vi "Layout FGV.vi"(7 "String":string, 8 "error in (no error)":errorcluster, 11 "InitRef":T5) -> (0 "error out":errorcluster)   [LabVIEW 2020, in "MDI ViewManager.lvlib"]
uses:
  MDI ViewManager.lvlib
  <vilib>/Utility/miscctls.llb/LVPositionTypeDef.ctl
  <vilib>/Utility/miscctls.llb/LVBoundsTypeDef.ctl
  <vilib>/Utility/miscctls.llb/LVPointTypeDef.ctl
  Typedef/Update ViewList.ctl
  Typedef/LayoutMap.ctl
panel:
  in  "map in":map{string, T1}(c390)
  in  "Variant":variant
  in  "name":string
  in  "file (use dialog)":path
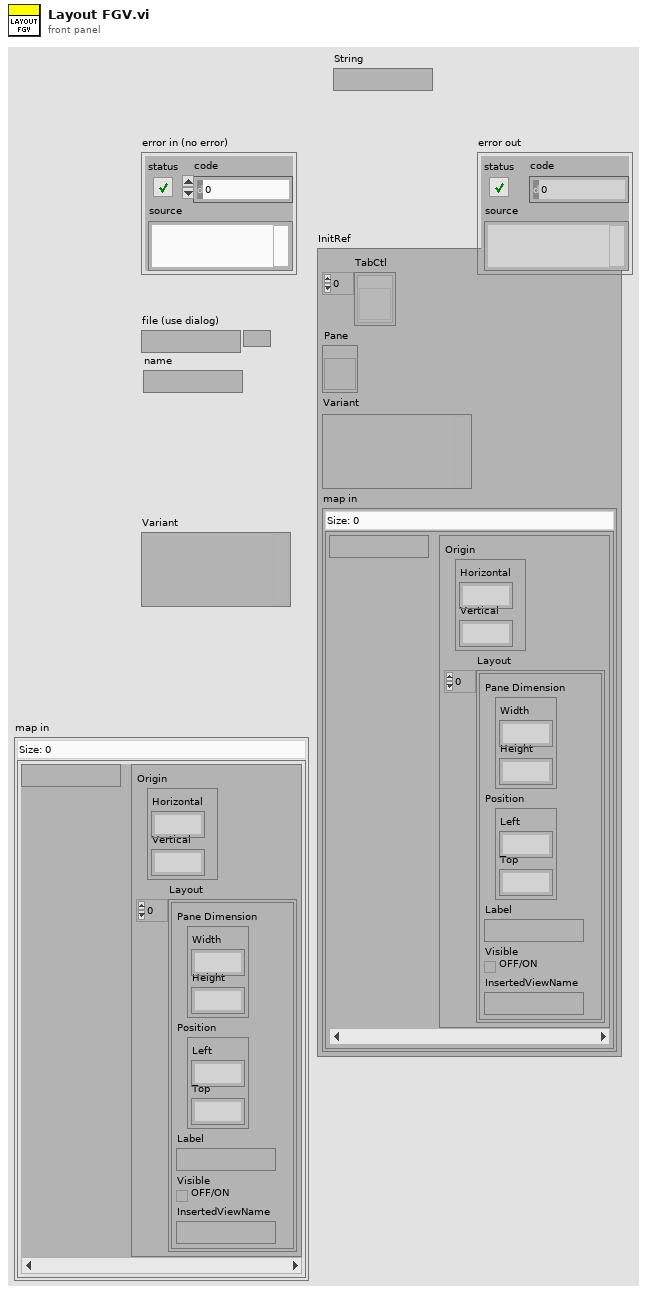
[diagram p1: front panel]
types:
  T1 = typedef "MDI ViewManager.lvlib/LayoutMap.ctl" = cluster{"Origin":T2, "Layout":cluster{"Pane Dimension":T3, "Position":T4, "Label":string, "Visible":bool, "InsertedViewName":string}[]}
  T2 = typedef "LVPointTypeDef.ctl" = cluster{"Horizontal":i16, "Vertical":i16}
  T3 = typedef "LVBoundsTypeDef.ctl" = cluster{"Width":u32, "Height":u32}
  T4 = typedef "LVPositionTypeDef.ctl" = cluster{"Left":i32, "Top":i32}
  T5 = cluster{"TabCtl":refnum<vi>[], "Pane":refnum<vi>, "Variant":variant, "map in":map{string, T1}}
  T6 = cluster{"Origin":T2, "Layout":cluster{"Pane Dimension":T3, "Position":T4, "Label":string, "Visible":bool, "InsertedViewName":string}[]}
  T7 = typedef "MDI ViewManager.lvlib/Update ViewList.ctl" = cluster{"Name":string, "VIPath":path, "Height(Default)":u32, "Widht(Default)":u32, "VIRef":refnum<vi>}
  T8 = cluster{"Pane Dimension":T3, "Position":T4, "Label":string, "Visible":bool, "InsertedViewName":string}
  T9 = cluster{"Pane Dimension":T3, "Position":T4, "Label":string, "Visible":bool, "InsertedViewName":string}[]
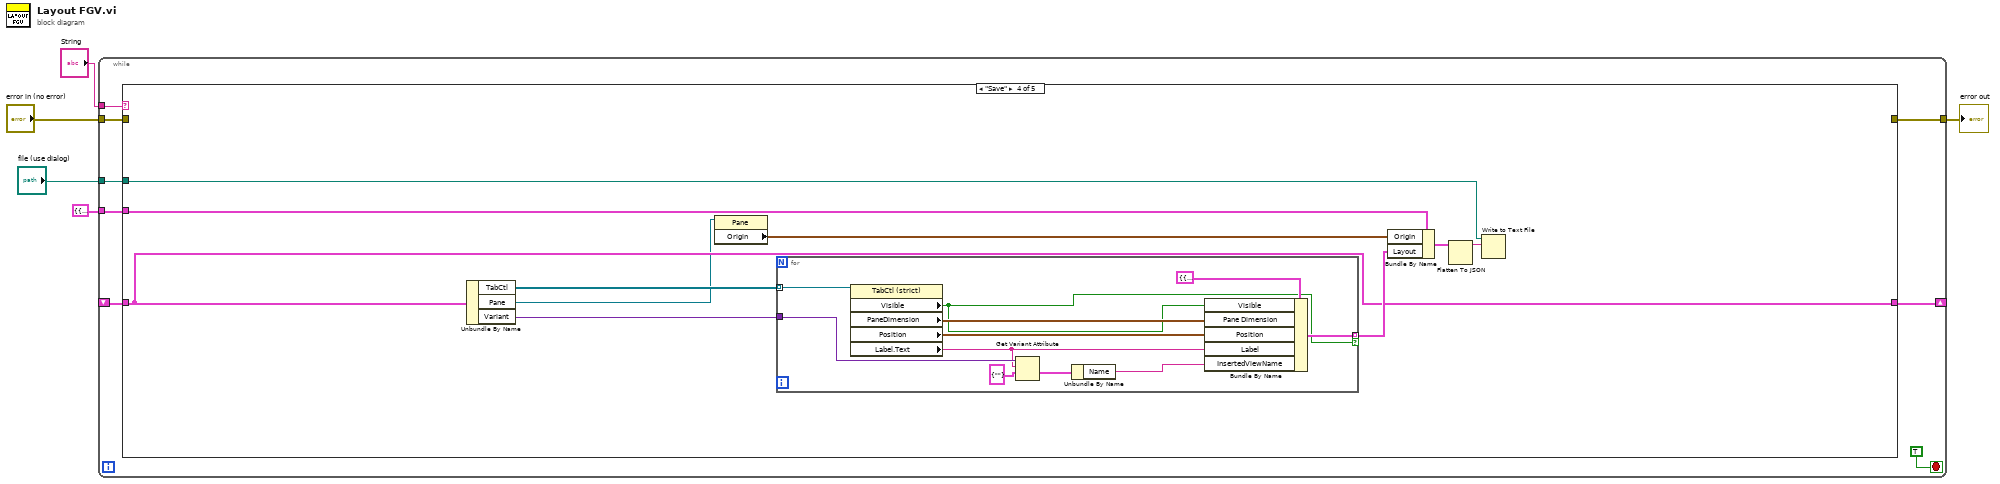
[diagram p0: block diagram]
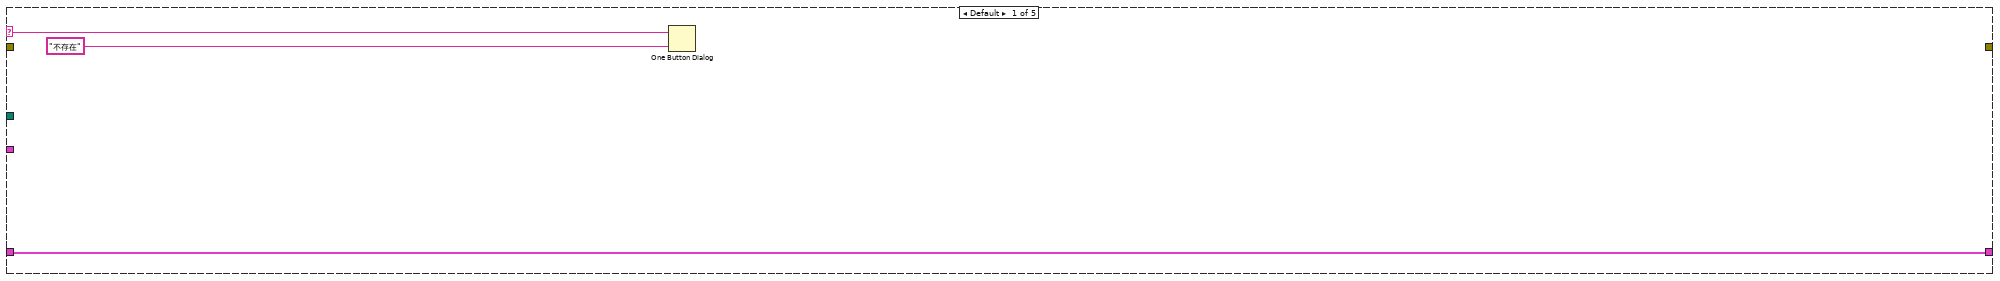
[diagram p2: hidden frame]
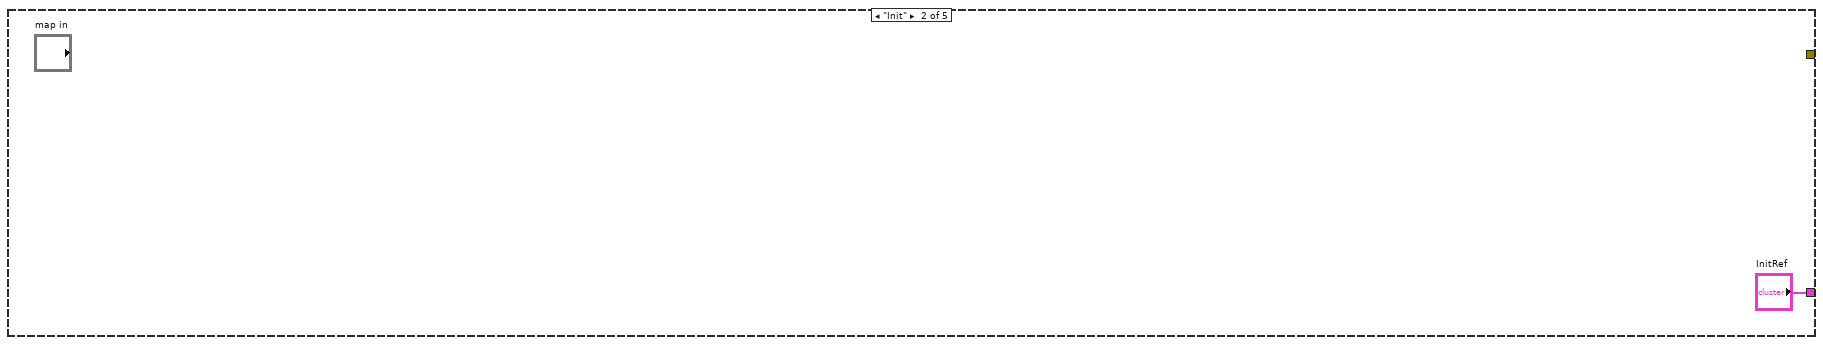
[diagram p3: hidden frame]
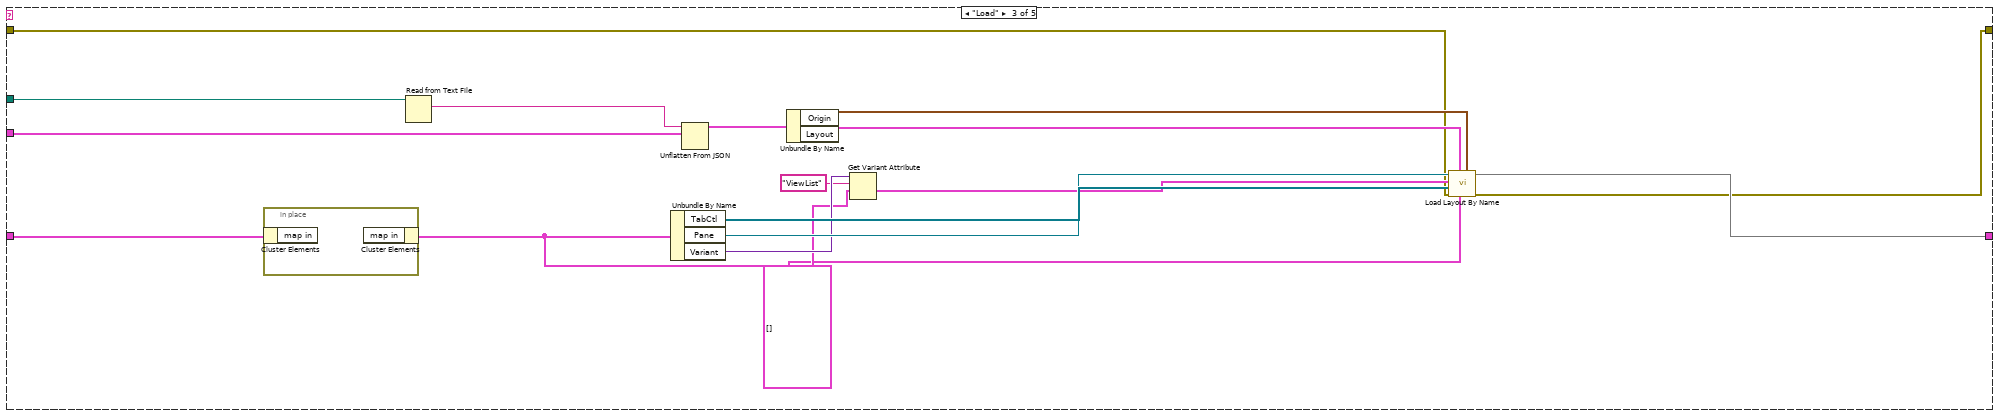
[diagram p4: hidden frame]
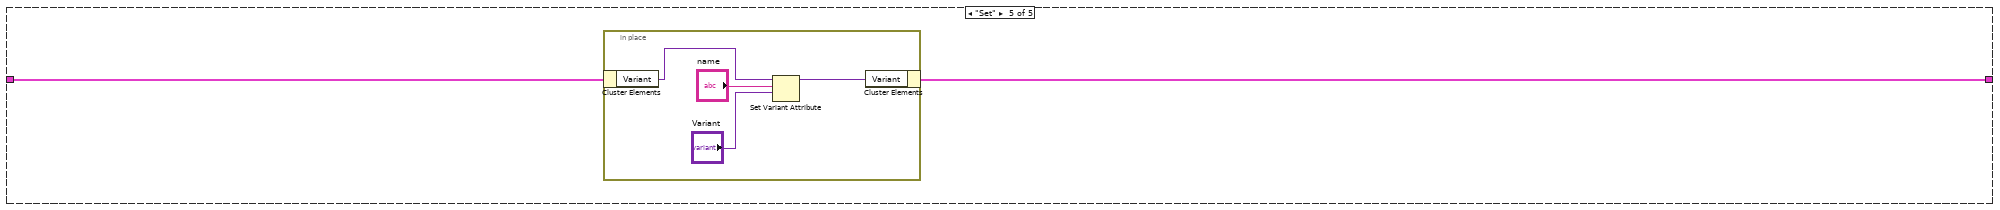
[diagram p5: hidden frame]
diagram:
  n1 = while {
    tunnel: "String" -> [w11]
    tunnel: "file (use dialog)" -> [w10]
    shift-right: [w9] -> _
    shift-left: _ -> [w12]
    tunnel: T6 {"Origin"={"Horizontal"=0, "Vertical"=0}, "Layout"=[]} -> [w8]
    tunnel: "error in (no error)" -> [w7]
    tunnel: [w6] -> w1
    stop <- TRUE stop-if-true
    n2 = case shown="\"Save\"" w11 {
      selector: w11 -> [w15 _ _ _ _]
      tunnel: w12 -> [w16 _ w23 w38 w57]
      tunnel: w10 -> [_ _ w33 w43 _]
      tunnel: [w16 "InitRef" w22 w38 w56] -> w9
      tunnel: w8 -> [_ _ w32 w39 _]
      tunnel: w7 -> [_ _ w20 _ _]
      tunnel: [_ _ w19 _ _] -> w6
      frame Default {
        n3 = One Button Dialog(message=w15, button name ("OK")="不存在") -> ()  [unwired: 1 out]
      }
      frame "Init" {
      }
      frame "Load" {
        n4 = in-place {
          n5 = in-place-cluster #1(w23) -> ()  [unwired: 1 out]
          n6 = in-place-cluster #1() -> (w18:T5)  [unwired: 1 in]
        }
        n7 = Read from Text File(file (use dialog)=w33) -> (text=w34:string)  [unwired: 3 in, 3 out]
        n8 = Unbundle By Name(w18) -> ("TabCtl"=w29:refnum<vi>[], "Pane"=w28:refnum<vi>, "Variant"=w26:variant)
        n9 = Unflatten From JSON(JSON string=w34, type and defaults=w32) -> (value=w31:T6)  [unwired: 5 in, 1 out]
        n10 = Unbundle By Name(w31) -> ("Origin"=w27:T2, "Layout"=w30:T9)
        n11 = Get Variant Attribute(Variant=w26, name="ViewList", default value (empty Variant)=T7[] [] ("1.Val.UpdateInsertableVI")) -> (value=w21:T7[])  [unwired: 1 in, 3 out]
        n12 = call "Load Layout By Name.vi"(5:w27, 6:w18, 7:w30, "error in (no error)"=w20, 9:w29, "key"=w21, "Cluster"=w28) -> ("error out"=w19:errorcluster, 3:w22)  [unwired: 3 in]
      }
      frame "Save" {
        n13 = Unbundle By Name(w38) -> ("TabCtl"=w37:refnum<vi>[], "Pane"=w36:refnum<vi>, "Variant"=w35:variant)
        n14 = property class="Pane"(reference=w36) -> ("Origin"=w42:T2)  [unwired: 1 in, 2 out]
        n15 = for {
          tunnel: w37 -> [w50] mode=indexing
          tunnel: [w53] -> w41 mode=indexing if=w51
          tunnel: w35 -> [w49]
          n16 = property class="TabCtl (strict)"(reference=w50) -> ("Visible"=w51:bool, "PaneDimension"=w55:T3, "Position"=w54:T4, "Label.Text"=w48:string)  [unwired: 1 in, 2 out]
          n17 = Get Variant Attribute(Variant=w49, name=w48, default value (empty Variant)=cluster{"Name":string} {"Name"=""} ("output cluster")) -> (value=w46:cluster{"Name":string})  [unwired: 1 in, 3 out]
          n18 = Unbundle By Name(w46) -> ("Name"=w45:string)
          n19 = Bundle By Name(cluster=T8 {"Pane Dimension"={"Width"=0, "Height"=0}, "Position"={"Left"=0, "Top"=0}, "Label"="", "Visible"=FALSE, "InsertedViewName"=""}, "Visible"=w51, "Pane Dimension"=w55, "Position"=w54, "Label"=w48, "InsertedViewName"=w45) -> (w53:T8)
        }
        n20 = Bundle By Name(cluster=w39, "Origin"=w42, "Layout"=w41) -> (w40:T6)
        n21 = Flatten To JSON(anything=w40) -> (JSON string=w44:string)  [unwired: 2 in, 1 out]
        n22 = Write to Text File(file (use dialog)=w43, text=w44) -> ()  [unwired: 2 in, 3 out]
      }
      frame "Set" {
        n23 = in-place {
          n24 = in-place-cluster #2(w57) -> ("Variant"=w61:variant)
          n25 = Set Variant Attribute(Variant=w61, name="name", value="Variant") -> (Variant out=w60:variant)  [unwired: 1 in, 2 out]
          n26 = in-place-cluster #2("Variant"=w60) -> (w56:T5)
        }
      }
    }
  }
  "error out" <- w1
